vi "Insert into Subpanel.vi"(8 "error in (no error)":errorcluster, 9 "Sub Panel":refnum<vi>, 10 "Panel":refnum<class "Panel.lvclass">, 11 "PanelManager in":refnum<class "PanelManager.lvclass">) -> (0 "error out":errorcluster, 1 "Replaced?":bool, 2 "Replaced Panel":refnum<class "Panel.lvclass">, 3 "PanelManager out":refnum<class "PanelManager.lvclass">)   [LabVIEW 2018, in "OOPanel.lvlib" / "PanelManager.lvclass"]
uses:
  PanelManager.lvclass
  Panel/Panel.lvclass
  Panel/State.ctl
  PanelManager.lvclass/PanelManager.ctl
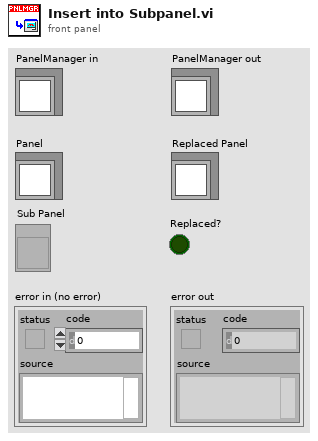
[diagram p1: front panel]
types:
  T1 = typedef "OOPanel.lvlib/Panel.lvclass/State.ctl" = enum16{"Idle", "Hidden", "Visible", "Subpanel"}
  T2 = typedef "OOPanel.lvlib/PanelManager.lvclass/Ref Data.ctl" = cluster{"Panels":T3, "Subpanel Map":T4}
  T3 = typedef "OOPanel.lvlib/PanelManager.lvclass/Panels.ctl" = cluster{"Names":string[], "Instances":refnum<class "Panel.lvclass">[]}
  T4 = typedef "OOPanel.lvlib/PanelManager.lvclass/SubPanel Map.ctl" = cluster{"SubPanels":refnum<vi>[], "Panels":refnum<class "Panel.lvclass">[]}
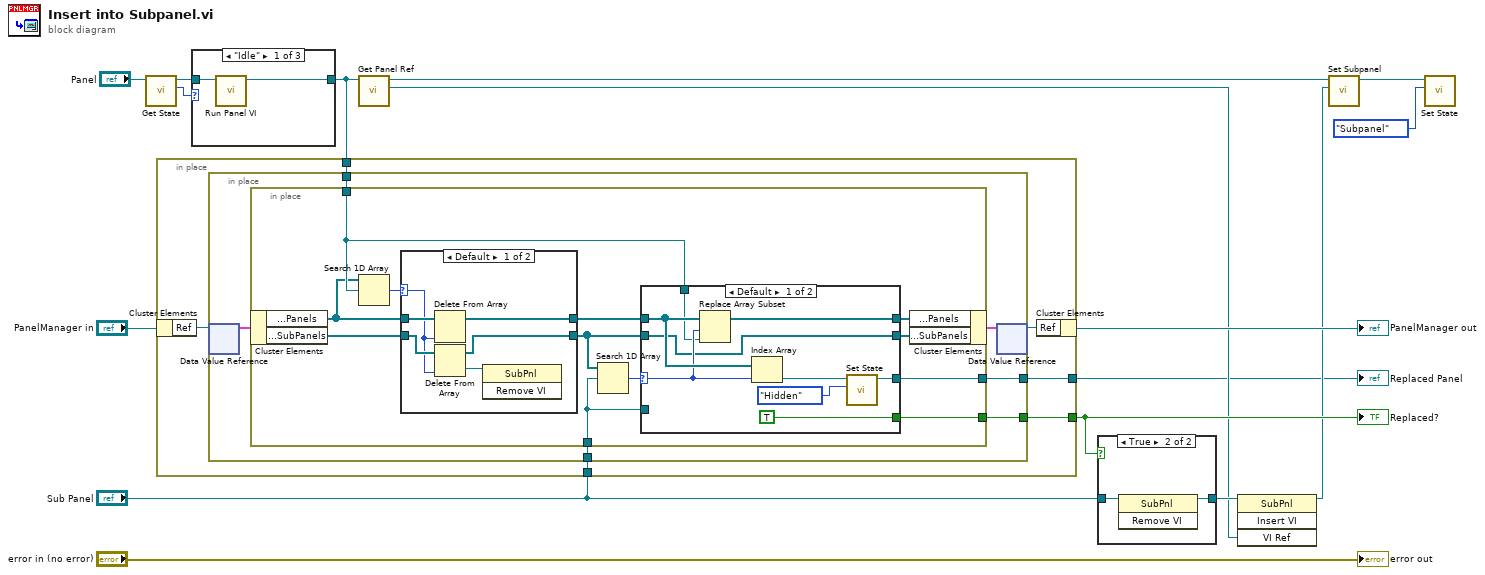
[diagram p0: block diagram]
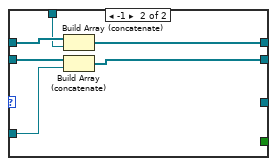
[diagram p3: hidden frame]
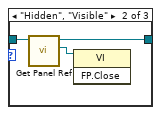
[diagram p4: hidden frame]
diagram:
  n1 = call "Get State.vi"("Panel in"="Panel") -> ("State"=w9:T1, "Panel out"=w10:refnum<class "Panel.lvclass">)  [unwired: 8 in, 1 out]
  n2 = case shown="\"Idle\"" w9 {
    tunnel: w10 -> [w18 w21 w22]
    tunnel: [w17 w19 w22] -> w7
    frame "Idle" {
      n3 = call "Run Panel VI.vi"("Panel in"=w18) -> ("Panel out"=w17:refnum<class "Panel.lvclass">)  [unwired: 9 in, 1 out]
    }
    frame "Hidden", "Visible" {
      n4 = call "Get Panel Ref.vi"("Panel in"=w21) -> ("Panel Ref"=w20:refnum<vi>, "Panel out"=w19:refnum<class "Panel.lvclass">)  [unwired: 8 in, 1 out]
      n5 = invoke class="VI" method="FP.Close"(reference=w20) -> ()  [unwired: 2 in, 3 out]
    }
    frame "Subpanel" {
    }
  }
  n6 = in-place {
    in-place-border: "Sub Panel" -> [w28]
    in-place-border: w7 -> [w25]
    in-place-border: [w24] -> w3
    in-place-border: [w23] -> w14
    n7 = in-place-cluster #1("PanelManager in") -> ("Ref"=w27:refnum<data-value>)
    n8 = in-place {
      in-place-border: w28 -> [w32]
      in-place-border: w25 -> [w31]
      in-place-border: [w30] -> w24
      in-place-border: [w29] -> w23
      n9 = in-place-dvr #2(w27) -> (w34:T2)  [unwired: 1 out]
      n10 = in-place {
        in-place-border: w32 -> [w45]
        in-place-border: w31 -> [w40]
        in-place-border: [w42] -> w30
        in-place-border: [w41] -> w29
        n11 = in-place-cluster #3(w34) -> ("Subpanel Map.Panels"=w38:refnum<class "Panel.lvclass">[], "Subpanel Map.SubPanels"=w36:refnum<vi>[])
        n12 = Search 1D Array(1D array=w38, element=w40) -> (index of element=w39:i32)  [unwired: 1 in]
        n13 = case shown="Default" w39 {
          selector: w39 -> [w50 _]
          tunnel: w38 -> [w51 w54]
          tunnel: [w49 w54] -> w37
          tunnel: w36 -> [w52 w53]
          tunnel: [w48 w53] -> w35
          frame Default {
            n14 = Delete From Array(array=w51, index=w50) -> (array with subset deleted=w49:refnum<class "Panel.lvclass">[])  [unwired: 1 in, 1 out]
            n15 = Delete From Array(array=w52, index=w50) -> (deleted portion=w47:refnum<vi>, array with subset deleted=w48:refnum<vi>[])  [unwired: 1 in]
            n16 = invoke class="SubPnl" method="Remove VI"(reference=w47) -> ()  [unwired: 2 in, 3 out]
          }
          frame -1 {
          }
        }
        n17 = Search 1D Array(1D array=w35, element=w45) -> (index of element=w46:i32)  [unwired: 1 in]
        n18 = case shown="Default" w46 {
          selector: w46 -> [w62 _]
          tunnel: w35 -> [w59 w66]
          tunnel: w45 -> [_ w65]
          tunnel: w37 -> [w63 w69]
          tunnel: w40 -> [w61 w68]
          tunnel: [w60 w67] -> w44
          tunnel: [w59 w64] -> w43
          tunnel: [w55 _] -> w42
          tunnel: [TRUE _] -> w41
          frame Default {
            n19 = Replace Array Subset(array=w63, new element=w61, index=w62) -> (w60:refnum<class "Panel.lvclass">[])
            n20 = Index Array(array=w63, index=w62) -> (element=w56:refnum<class "Panel.lvclass">)
            n21 = call "Set State.vi"("State"=State."Hidden", "Panel in"=w56) -> ("Panel out"=w55:refnum<class "Panel.lvclass">)  [unwired: 8 in, 1 out]
          }
          frame -1 {
            n22 = Build Array (concatenate)(w69, w68) -> (w67:refnum<class "Panel.lvclass">[])
            n23 = Build Array (concatenate)(w66, w65) -> (w64:refnum<vi>[])
          }
        }
        n24 = in-place-cluster #3("Subpanel Map.Panels"=w44, "Subpanel Map.SubPanels"=w43) -> (w33:T2)
      }
      n25 = in-place-dvr #2(w33) -> (w26:refnum<data-value>)  [unwired: 1 out]
    }
    n26 = in-place-cluster #1("Ref"=w26) -> (→"PanelManager out":refnum<class "PanelManager.lvclass">)
  }
  "Replaced Panel" <- w3
  "Replaced?" <- w14
  n27 = call "Get Panel Ref.vi"("Panel in"=w7) -> ("Panel Ref"=w6:refnum<vi>, "Panel out"=w4:refnum<class "Panel.lvclass">)  [unwired: 8 in, 1 out]
  n28 = case shown="True" w14 {
    tunnel: "Sub Panel" -> [w70 w72]
    tunnel: [w70 w71] -> w12
    frame False {
    }
    frame True {
      n29 = invoke class="SubPnl" method="Remove VI"(reference=w72) -> (reference out=w71:refnum<vi>)  [unwired: 2 in, 2 out]
    }
  }
  n30 = invoke class="SubPnl" method="Insert VI"(reference=w12, "VI Ref"=w6) -> (reference out=w5:refnum<vi>)  [unwired: 2 in, 3 out]
  n31 = call "Set Subpanel.vi"("Subpanel"=w5, "Panel in"=w4) -> ("Panel out"=w1:refnum<class "Panel.lvclass">)  [unwired: 8 in, 1 out]
  n32 = call "Set State.vi"("State"=State."Subpanel", "Panel in"=w1) -> ()  [unwired: 8 in, 2 out]
  "error out" <- "error in (no error)"
